vi "initAD.vi"() -> (0 "待读取数据长度":i32, 1 "采样频率":dbl, 2 "设备":dbl)   [LabVIEW 2018]
uses:
  main/PCI8552B_32.dll
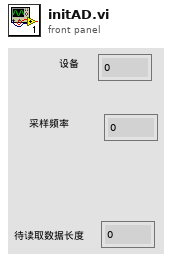
[diagram p1: front panel]
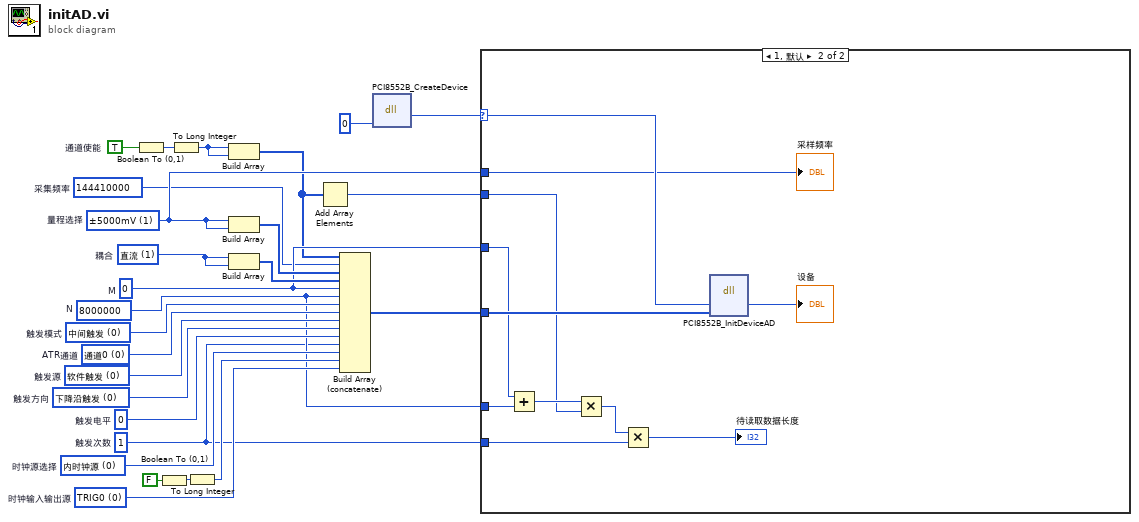
[diagram p0: block diagram]
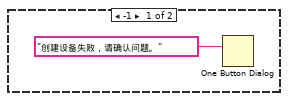
[diagram p2: hidden frame]
diagram:
  w6 = 8000000  # N
  w7 = 0  # M
  w8 = 1 items=["交流", "直流"]  # 耦合
  w3 = 1 items=["±1000mV", "±5000mV"]  # 量程选择
  w10 = TRUE  # 通道使能
  w1 = 144410000  # 采集频率
  w15 = 0 items=["中间触发", "后触发", "预触发", "硬件延时触发"]  # 触发模式
  w13 = 0 items=["通道0", "通道1"]  # ATR通道
  w24 = 0 items=["软件触发", "DTR作为触发源", "ATR作为触发源", "Trigger信号触发"]  # 触发源
  w23 = 0 items=["下降沿触发", "上升沿触发", "上下边沿均触发", ""]  # 触发方向
  w22 = 0  # 触发电平
  w4 = 1  # 触发次数
  w20 = 0 items=["TRIG0", "TRIG1", "TRIG2", "TRIG3"]  # 时钟输入输出源
  w21 = 0 items=["内时钟源", "主卡10M时钟源", "外部时钟"]  # 时钟源选择
  n1 = Boolean To (0,1)(Boolean=w10) -> (0, 1=w17:i16)
  n2 = Boolean To (0,1)(Boolean=FALSE ("主设备使能")) -> (0, 1=w18:i16)
  n3 = To Long Integer(number=w17) -> (32bit integer=w9:i32)
  n4 = To Long Integer(number=w18) -> (32bit integer=w19:i32)
  n5 = Build Array(w9, w9) -> (w2:i32[])
  n6 = Build Array(w3, w3) -> (w14:i32[])
  n7 = Build Array(w8, w8) -> (w25:i32[])
  n8 = Add Array Elements(numeric array=w2) -> (sum=w5:i32)
  n9 = Build Array (concatenate)(w2, w1, w14, w25, w7, w6, w15, w13, w24, w23, w22, w4, w21, w19, w20) -> (w16:i32[])
  n10 = dll-call lib="PTH2…abs E\nPersonal Fileç ”ç©¶ç”Ÿå­¦ä¹ 202002-202007ç ”ä¸€ä¸‹å­¦æœŸwork2020\nSARControllerSAR-ControllermainPCI8552B_32.dll" fn="PCI8552B_CreateDevice" label="CreateDevice"("DeviceLgcID"=0) -> ("返回类型"=w11:i32)  [unwired: 4 in, 2 out]
  n11 = case shown="1, 默认" w11 {
    selector: w11 -> [_ w30]
    tunnel: w16 -> [_ w38]
    tunnel: w7 -> [_ w37]
    tunnel: w6 -> [_ w36]
    tunnel: w5 -> [_ w34]
    tunnel: w4 -> [_ w32]
    tunnel: w3 -> [_ w28]
    frame -1 {
      n12 = One Button Dialog(message="创建设备失败，请确认问题。") -> ()  [unwired: 1 in, 1 out]
    }
    frame 1, Default {
      n13 = Add(x=w37, y=w36) -> (x+y=w35:i32)
      n14 = Multiply(x=w35, y=w34) -> (x*y=w33:i32)
      n15 = Multiply(x=w33, y=w32) -> (x*y=→"待读取数据长度":i32)
      n16 = dll-call lib="PTH2…abs E\nPersonal Fileç ”ç©¶ç”Ÿå­¦ä¹ 202002-202007ç ”ä¸€ä¸‹å­¦æœŸwork2020\nSARControllerSAR-ControllermainPCI8552B_32.DLL" fn="PCI8552B_InitDeviceAD" label="InitDeviceAD"("hDevice"=w30, "pADPara"=w38) -> ("hDevice"=→"设备":i32)  [unwired: 5 in, 2 out]
      "采样频率" <- w28
    }
  }
